vi "TalonFXSConfigurator.vi"(6 "timeoutSeconds":dbl=0.05, 8 "error in":errorcluster, 10 "DeviceConfiguration":T2={"Future Proof Configs"=FALSE, "MotorOutputInverted"=0, "MotorOutputNeutralMode"=0, "MotorOutputDutyCycleNeutralDeadband"=0.0, "MotorOutputPeakForwardDutyCycle"=1.0, "MotorOutputPeakReverseDutyCycle"=-1.0, "MotorOutputControlTimesyncFreqHz"=0.0, "CurrentLimitsStatorCurrentLimit"=120.0, "CurrentLimitsStatorCurrentLimitEnable"=TRUE, "CurrentLimitsSupplyCurrentLimit"=70.0, "CurrentLimitsSupplyCurrentLimitEnable"=TRUE, "CurrentLimitsSupplyCurrentLowerLimit"=40.0, "CurrentLimitsSupplyCurrentLowerTime"=1.0, "VoltageSupplyVoltageTimeConstant"=0.0, "VoltagePeakForwardVoltage"=16.0, "VoltagePeakReverseVoltage"=-16.0, "ExternalFeedbackSensorToMechanismRatio"=1.0, "ExternalFeedbackRotorToSensorRatio"=1.0, "ExternalFeedbackFeedbackRemoteSensorID"=0, "ExternalFeedbackVelocityFilterTimeConstant"=0.0, "ExternalFeedbackAbsoluteSensorOffset"=0.0, "ExternalFeedbackExternalFeedbackSensorSource"=0, "ExternalFeedbackSensorPhase"=0, "ExternalFeedbackQuadratureEdgesPerRotation"=4096, "ExternalFeedbackAbsoluteSensorDiscontinuityPoint"=0.5, "DifferentialSensorsDifferentialSensorSource"=0, "DifferentialSensorsDifferentialTalonFXSensorID"=0, "DifferentialSensorsDifferentialRemoteSensorID"=0, "DifferentialSensorsSensorToDifferentialRatio"=1.0, "DifferentialConstantsPeakDifferentialDutyCycle"=1.0, "DifferentialConstantsPeakDifferentialVoltage"=16.0, "DifferentialConstantsPeakDifferentialTorqueCurrent"=800.0, "OpenLoopRampsDutyCycleOpenLoopRampPeriod"=0.0, "OpenLoopRampsVoltageOpenLoopRampPeriod"=0.0, "OpenLoopRampsTorqueOpenLoopRampPeriod"=0.0, "ClosedLoopRampsDutyCycleClosedLoopRampPeriod"=0.0, "ClosedLoopRampsVoltageClosedLoopRampPeriod"=0.0, "ClosedLoopRampsTorqueClosedLoopRampPeriod"=0.0, "HardwareLimitSwitchForwardLimitType"=0, "HardwareLimitSwitchForwardLimitAutosetPositionEnable"=FALSE, "HardwareLimitSwitchForwardLimitAutosetPositionValue"=0.0, "HardwareLimitSwitchForwardLimitEnable"=TRUE, "HardwareLimitSwitchForwardLimitSource"=0, "HardwareLimitSwitchForwardLimitRemoteSensorID"=0, "HardwareLimitSwitchReverseLimitType"=0, "HardwareLimitSwitchReverseLimitAutosetPositionEnable"=FALSE, "HardwareLimitSwitchReverseLimitAutosetPositionValue"=0.0, "HardwareLimitSwitchReverseLimitEnable"=TRUE, "HardwareLimitSwitchReverseLimitSource"=0, "HardwareLimitSwitchReverseLimitRemoteSensorID"=0, "AudioBeepOnBoot"=TRUE, "AudioBeepOnConfig"=TRUE, "AudioAllowMusicDurDisable"=FALSE, "SoftwareLimitSwitchForwardSoftLimitEnable"=FALSE, "SoftwareLimitSwitchReverseSoftLimitEnable"=FALSE, "SoftwareLimitSwitchForwardSoftLimitThreshold"=0.0, "SoftwareLimitSwitchReverseSoftLimitThreshold"=0.0, "MotionMagicMotionMagicCruiseVelocity"=0.0, "MotionMagicMotionMagicAcceleration"=0.0, "MotionMagicMotionMagicJerk"=0.0, "MotionMagicMotionMagicExpo_kV"=0.12, "MotionMagicMotionMagicExpo_kA"=0.1, "CustomParamsCustomParam0"=0, "CustomParamsCustomParam1"=0, "ClosedLoopGeneralContinuousWrap"=FALSE, "ClosedLoopGeneralDifferentialContinuousWrap"=FALSE, "ClosedLoopGeneralGainSchedErrorThreshold"=0.0, "ClosedLoopGeneralGainSchedKpBehavior"=0, "CommutationAdvancedHallSupport"=0, "CommutationMotorArrangement"=0, "CommutationBrushedMotorWiring"=0, "CustomBrushlessMotorMotorKv"=500.0, "CustomBrushlessMotorPolePairCount"=1, "CustomBrushlessMotorHallDuringAB"=0, "CustomBrushlessMotorHallDuringAC"=0, "CustomBrushlessMotorHallCCWSelect"=FALSE, "CustomBrushlessMotorHallDirection"=FALSE, "ExternalTempThermistorMaxTemperature"=0.0, "ExternalTempThermistorBeta"=0.0, "ExternalTempThermistorR0"=0.0, "ExternalTempTempSensorRequired"=0, "Slot0kP"=0.0, "Slot0kI"=0.0, "Slot0kD"=0.0, "Slot0kS"=0.0, "Slot0kV"=0.0, "Slot0kA"=0.0, "Slot0kG"=0.0, "Slot0GravityType"=0, "Slot0StaticFeedforwardSign"=0, "Slot0GravityArmPositionOffset"=0.0, "Slot0GainSchedBehavior"=0, "Slot1kP"=0.0, "Slot1kI"=0.0, "Slot1kD"=0.0, "Slot1kS"=0.0, "Slot1kV"=0.0, "Slot1kA"=0.0, "Slot1kG"=0.0, "Slot1GravityType"=0, "Slot1StaticFeedforwardSign"=0, "Slot1GravityArmPositionOffset"=0.0, "Slot1GainSchedBehavior"=0, "Slot2kP"=0.0, "Slot2kI"=0.0, "Slot2kD"=0.0, "Slot2kS"=0.0, "Slot2kV"=0.0, "Slot2kA"=0.0, "Slot2kG"=0.0, "Slot2GravityType"=0, "Slot2StaticFeedforwardSign"=0, "Slot2GravityArmPositionOffset"=0.0, "Slot2GainSchedBehavior"=0} {"MotorOutputInverted" items=["CounterClockwise_Positive", "Clockwise_Positive"]; "MotorOutputNeutralMode" items=["Coast", "Brake"]; "ExternalFeedbackExternalFeedbackSensorSource" items=["Commutation", "RemoteCANcoder", "RemotePigeon2Yaw", "RemotePigeon2Pitch", "RemotePigeon2Roll", "FusedCANcoder", "SyncCANcoder", "Quadrature", "PulseWidth", "RemoteCANdiPWM1", "RemoteCANdiPWM2", "RemoteCANdiQuadrature", "FusedCANdiPWM1", "FusedCANdiPWM2", "FusedCANdiQuadrature", "SyncCANdiPWM1", "SyncCANdiPWM2"]; "ExternalFeedbackSensorPhase" items=["Aligned", "Opposed"]; "DifferentialSensorsDifferentialSensorSource" items=["Disabled", "RemoteTalonFX_HalfDiff", "RemotePigeon2Yaw", "RemotePigeon2Pitch", "RemotePigeon2Roll", "RemoteCANcoder", "RemoteCANdiPWM1", "RemoteCANdiPWM2", "RemoteCANdiQuadrature"]; "HardwareLimitSwitchForwardLimitType" items=["NormallyOpen", "NormallyClosed"]; "HardwareLimitSwitchForwardLimitSource" items=["LimitSwitchPin"=0, "RemoteTalonFX"=1, "RemoteCANifier"=2, "RemoteCANcoder"=4, "RemoteCANrange"=6, "RemoteCANdiS1"=7, "RemoteCANdiS2"=8, "Disabled"=3]; "HardwareLimitSwitchReverseLimitType" items=["NormallyOpen", "NormallyClosed"]; "HardwareLimitSwitchReverseLimitSource" items=["LimitSwitchPin"=0, "RemoteTalonFX"=1, "RemoteCANifier"=2, "RemoteCANcoder"=4, "RemoteCANrange"=6, "RemoteCANdiS1"=7, "RemoteCANdiS2"=8, "Disabled"=3]; "ClosedLoopGeneralGainSchedKpBehavior" items=["Continuous", "Discontinuous"]; "CommutationAdvancedHallSupport" items=["Disabled", "Enabled"]; "CommutationMotorArrangement" items=["Disabled"=0, "Minion_JST"=1, "Brushed_DC"=2, "NEO_JST"=5, "NEO550_JST"=6, "VORTEX_JST"=7, "Custom Brushless"=8]; "CommutationBrushedMotorWiring" items=["Leads_A_and_B", "Leads_A_and_C", "Leads_B_and_C"]; "ExternalTempTempSensorRequired" items=["Required", "Not_Required"]; "Slot0GravityType" items=["Elevator_Static", "Arm_Cosine"]; "Slot0StaticFeedforwardSign" items=["UseVelocitySign", "UseClosedLoopSign"]; "Slot0GainSchedBehavior" items=["Inactive", "ZeroOutput", "UseSlot0", "UseSlot1", "UseSlot2"]; "Slot1GravityType" items=["Elevator_Static", "Arm_Cosine"]; "Slot1StaticFeedforwardSign" items=["UseVelocitySign", "UseClosedLoopSign"]; "Slot1GainSchedBehavior" items=["Inactive", "ZeroOutput", "UseSlot0", "UseSlot1", "UseSlot2"]; "Slot2GravityType" items=["Elevator_Static", "Arm_Cosine"]; "Slot2StaticFeedforwardSign" items=["UseVelocitySign", "UseClosedLoopSign"]; "Slot2GainSchedBehavior" items=["Inactive", "ZeroOutput", "UseSlot0", "UseSlot1", "UseSlot2"]}, 11 "DeviceReference":T1) -> (0 "error out":errorcluster)   [LabVIEW 2025]
uses:
  <vilib>/Rock Robotics/WPI/ThirdParty/Phoenix6/DeviceReference.ctl
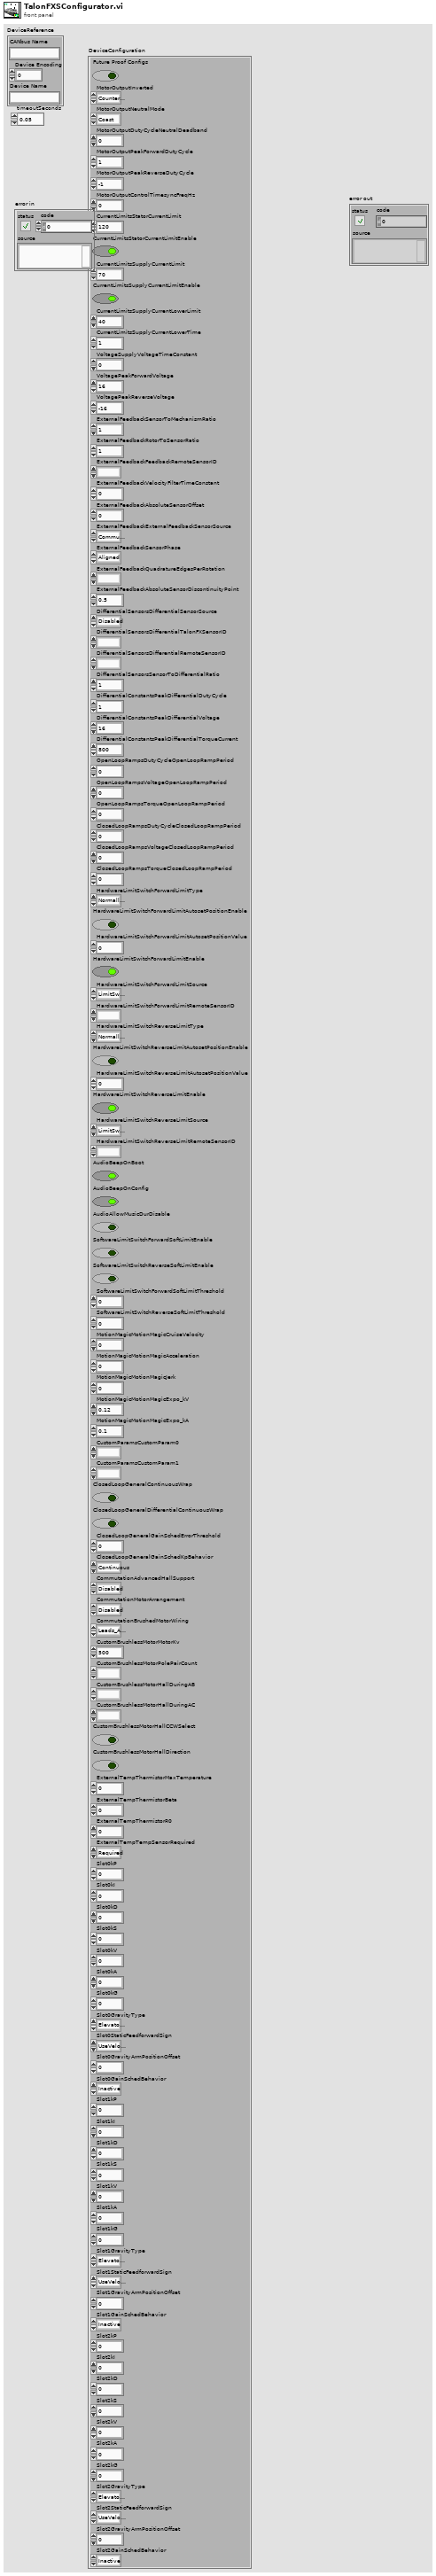
[diagram p1: front panel]
types:
  T1 = typedef "DeviceReference.ctl" = cluster{"CANbus Name":string, "Device Encoding":u32, "Device Name":string}
  T2 = cluster{"Future Proof Configs":bool, "MotorOutputInverted":u16, "MotorOutputNeutralMode":u16, "MotorOutputDutyCycleNeutralDeadband":dbl, "MotorOutputPeakForwardDutyCycle":dbl, "MotorOutputPeakReverseDutyCycle":dbl, "MotorOutputControlTimesyncFreqHz":dbl, "CurrentLimitsStatorCurrentLimit":dbl, "CurrentLimitsStatorCurrentLimitEnable":bool, "CurrentLimitsSupplyCurrentLimit":dbl, "CurrentLimitsSupplyCurrentLimitEnable":bool, "CurrentLimitsSupplyCurrentLowerLimit":dbl, "CurrentLimitsSupplyCurrentLowerTime":dbl, "VoltageSupplyVoltageTimeConstant":dbl, "VoltagePeakForwardVoltage":dbl, "VoltagePeakReverseVoltage":dbl, "ExternalFeedbackSensorToMechanismRatio":dbl, "ExternalFeedbackRotorToSensorRatio":dbl, "ExternalFeedbackFeedbackRemoteSensorID":u16, "ExternalFeedbackVelocityFilterTimeConstant":dbl, "ExternalFeedbackAbsoluteSensorOffset":dbl, "ExternalFeedbackExternalFeedbackSensorSource":u16, "ExternalFeedbackSensorPhase":u16, "ExternalFeedbackQuadratureEdgesPerRotation":u16, "ExternalFeedbackAbsoluteSensorDiscontinuityPoint":dbl, "DifferentialSensorsDifferentialSensorSource":u16, "DifferentialSensorsDifferentialTalonFXSensorID":u16, "DifferentialSensorsDifferentialRemoteSensorID":u16, "DifferentialSensorsSensorToDifferentialRatio":dbl, "DifferentialConstantsPeakDifferentialDutyCycle":dbl, "DifferentialConstantsPeakDifferentialVoltage":dbl, "DifferentialConstantsPeakDifferentialTorqueCurrent":dbl, "OpenLoopRampsDutyCycleOpenLoopRampPeriod":dbl, "OpenLoopRampsVoltageOpenLoopRampPeriod":dbl, "OpenLoopRampsTorqueOpenLoopRampPeriod":dbl, "ClosedLoopRampsDutyCycleClosedLoopRampPeriod":dbl, "ClosedLoopRampsVoltageClosedLoopRampPeriod":dbl, "ClosedLoopRampsTorqueClosedLoopRampPeriod":dbl, "HardwareLimitSwitchForwardLimitType":u16, "HardwareLimitSwitchForwardLimitAutosetPositionEnable":bool, "HardwareLimitSwitchForwardLimitAutosetPositionValue":dbl, "HardwareLimitSwitchForwardLimitEnable":bool, "HardwareLimitSwitchForwardLimitSource":u16, "HardwareLimitSwitchForwardLimitRemoteSensorID":u16, "HardwareLimitSwitchReverseLimitType":u16, "HardwareLimitSwitchReverseLimitAutosetPositionEnable":bool, "HardwareLimitSwitchReverseLimitAutosetPositionValue":dbl, "HardwareLimitSwitchReverseLimitEnable":bool, "HardwareLimitSwitchReverseLimitSource":u16, "HardwareLimitSwitchReverseLimitRemoteSensorID":u16, "AudioBeepOnBoot":bool, "AudioBeepOnConfig":bool, "AudioAllowMusicDurDisable":bool, "SoftwareLimitSwitchForwardSoftLimitEnable":bool, "SoftwareLimitSwitchReverseSoftLimitEnable":bool, "SoftwareLimitSwitchForwardSoftLimitThreshold":dbl, "SoftwareLimitSwitchReverseSoftLimitThreshold":dbl, "MotionMagicMotionMagicCruiseVelocity":dbl, "MotionMagicMotionMagicAcceleration":dbl, "MotionMagicMotionMagicJerk":dbl, "MotionMagicMotionMagicExpo_kV":dbl, "MotionMagicMotionMagicExpo_kA":dbl, "CustomParamsCustomParam0":u16, "CustomParamsCustomParam1":u16, "ClosedLoopGeneralContinuousWrap":bool, "ClosedLoopGeneralDifferentialContinuousWrap":bool, "ClosedLoopGeneralGainSchedErrorThreshold":dbl, "ClosedLoopGeneralGainSchedKpBehavior":u16, "CommutationAdvancedHallSupport":u16, "CommutationMotorArrangement":u16, "CommutationBrushedMotorWiring":u16, "CustomBrushlessMotorMotorKv":dbl, "CustomBrushlessMotorPolePairCount":u16, "CustomBrushlessMotorHallDuringAB":u16, "CustomBrushlessMotorHallDuringAC":u16, "CustomBrushlessMotorHallCCWSelect":bool, "CustomBrushlessMotorHallDirection":bool, "ExternalTempThermistorMaxTemperature":dbl, "ExternalTempThermistorBeta":dbl, "ExternalTempThermistorR0":dbl, "ExternalTempTempSensorRequired":u16, "Slot0kP":dbl, "Slot0kI":dbl, "Slot0kD":dbl, "Slot0kS":dbl, "Slot0kV":dbl, "Slot0kA":dbl, "Slot0kG":dbl, "Slot0GravityType":u16, "Slot0StaticFeedforwardSign":u16, "Slot0GravityArmPositionOffset":dbl, "Slot0GainSchedBehavior":u16, "Slot1kP":dbl, "Slot1kI":dbl, "Slot1kD":dbl, "Slot1kS":dbl, "Slot1kV":dbl, "Slot1kA":dbl, "Slot1kG":dbl, "Slot1GravityType":u16, "Slot1StaticFeedforwardSign":u16, "Slot1GravityArmPositionOffset":dbl, "Slot1GainSchedBehavior":u16, "Slot2kP":dbl, "Slot2kI":dbl, "Slot2kD":dbl, "Slot2kS":dbl, "Slot2kV":dbl, "Slot2kA":dbl, "Slot2kG":dbl, "Slot2GravityType":u16, "Slot2StaticFeedforwardSign":u16, "Slot2GravityArmPositionOffset":dbl, "Slot2GainSchedBehavior":u16}
  T3 = enum8{"<Null>", "I8", "I16", "I32", "I64", "U8", "U16", "U32", "U64", "SGL", "DBL", "EXT", "CSG", "CDB", "CXT", "0x0F", "0x10", "0x11", "0x12", "0x13", "0x14", "Enum U8", "Enum U16", "Enum U32", "Enum U64", "SGL PQ", "DBL PQ", "EXT PQ", "CSG PQ", "CDB PQ", "CXT PQ", "0x1F", "0x20", "Boolean", "0x22", "0x23", "0x24", "0x25", "0x26", "0x27", "0x28", "0x29", "0x2A", "0x2B", "0x2C", "0x2D", "0x2E", "0x2F", "String", "0x31", "Path", "Pict", "0x34", "0x35", "0x36", "DAQ", "0x38", "0x39", "0x3A", "0x3B", "0x3C", "0x3D", "0x3E", "0x3F", "Array", "0x41", "0x42", "0x43", "0x44", "0x45", "0x46", "0x47", "0x48", "0x49", "0x4A", "0x4B", "0x4C", "0x4D", "0x4E", "0x4F", "Cluster", "0x51", "0x52", "Variant", "Waveform", "0x55", "0x56", "0x57", "0x58", "0x59", "0x5A", "0x5B", "0x5C", "0x5D", "0x5E", "Fixed Point", "0x60", "0x61", "0x62", "0x63", "0x64", "0x65", "0x66", "0x67", "0x68", "0x69", "0x6A", "0x6B", "0x6C", "0x6D", "0x6E", "0x6F", "Refnum", "0x71", "0x72", "Set Collection", "Map Collection"}
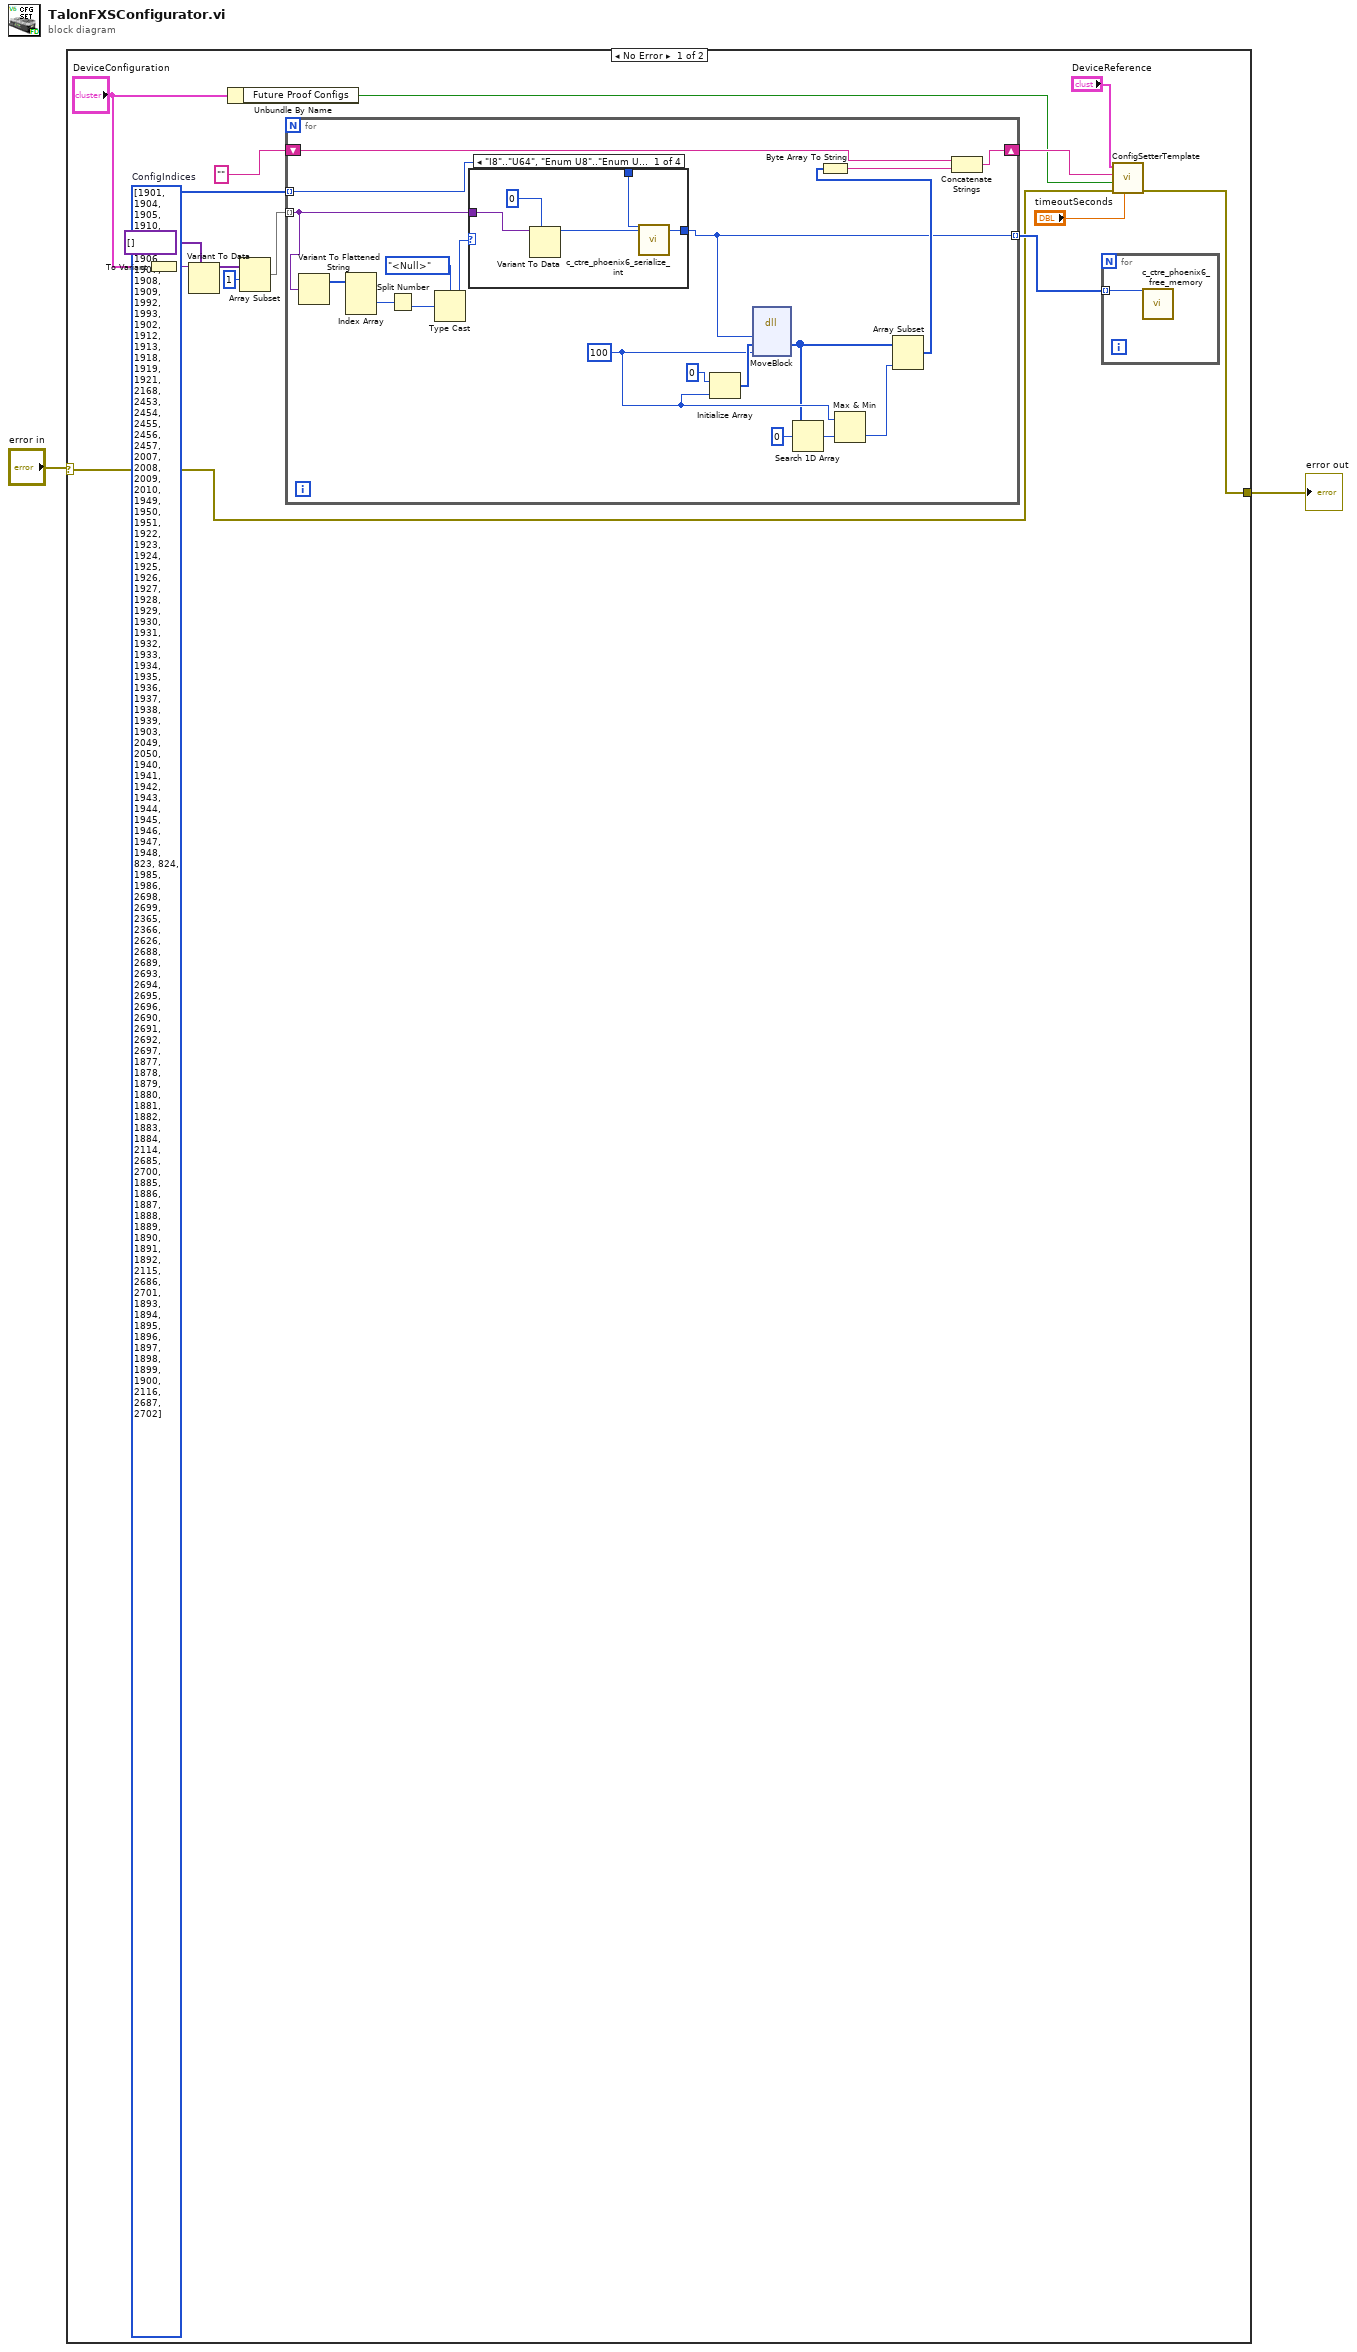
[diagram p0: block diagram]
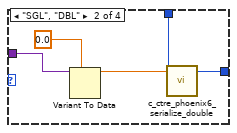
[diagram p2: hidden frame]
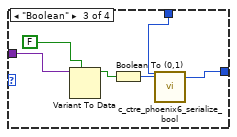
[diagram p3: hidden frame]
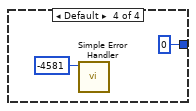
[diagram p4: hidden frame]
diagram:
  n1 = case shown="No Error" "error in" {
    selector: "error in" -> [w8 w56]
    tunnel: [w7 w56] -> w1
    frame No Error {
      w10 = i32[] [1901, 1904, 1905, 1910, 1911, 2167, 1906, 1907, 1908, 1909, 1992, 1993, 1902, 1912, 1913, 1918, 1919, 1921, 2168, 2453, 2454, 2455, 2456, 2457, 2007, 2008, 2009, 2010, 1949, 1950, 1951, 1922, 1923, 1924, 1925, 1926, 1927, 1928, 1929, 1930, 1931, 1932, 1933, 1934, 1935, 1936, 1937, 1938, 1939, 1903, 2049, 2050, 1940, 1941, 1942, 1943, 1944, 1945, 1946, 1947, 1948, 823, 824, 1985, 1986, 2698, 2699, 2365, 2366, 2626, 2688, 2689, 2693, 2694, 2695, 2696, 2690, 2691, 2692, 2697, 1877, 1878, 1879, 1880, 1881, 1882, 1883, 1884, 2114, 2685, 2700, 1885, 1886, 1887, 1888, 1889, 1890, 1891, 1892, 2115, 2686, 2701, 1893, 1894, 1895, 1896, 1897, 1898, 1899, 1900, 2116, 2687, 2702]  # ConfigIndices
      n2 = To Variant(anything="DeviceConfiguration") -> (Variant=w6:variant)
      n3 = Variant To Data(type=variant[] [], Variant=w6) -> (data=w3:variant[])  [unwired: 1 in, 1 out]
      n4 = Unbundle By Name("DeviceConfiguration") -> ("Future Proof Configs"=w9:bool)
      n5 = Array Subset(array=w3, index=1) -> (w12:variant[])  [unwired: 1 in]
      n6 = for {
        tunnel: w12 -> [w19] mode=indexing
        shift-right: [w35] -> w16
        shift-left: "" -> [w36]
        tunnel: [w24] -> w11 mode=indexing
        tunnel: w10 -> [w25] mode=indexing
        w28 = i64 100 ("size")
        n7 = Variant To Flattened String(Variant=w19) -> (1:w22:i16[])  [unwired: 1 out]
        n8 = Index Array(array=w22) -> (element #2=w23:i16)  [unwired: 3 in, 2 out]
        n9 = Split Number(x=w23) -> (lo(x)=w20:u8)  [unwired: 1 out]
        n10 = Type Cast(type=T3."<Null>", x=w20) -> (*(type *) &x=w18:T3)
        n11 = case shown="\"I8\"..\"U64\", \"Enum U8\"..\"Enum U64\"" w18 {
          tunnel: w19 -> [w41 w46 w52 _]
          tunnel: w25 -> [w39 w43 w48 _]
          tunnel: [w37 w42 w47 u32 0 ("Numeric 4")] -> w24
          frame "I8".."U64", "Enum U8".."Enum U64" {
            n12 = Variant To Data(type=0, Variant=w41) -> (data=w38:i32)  [unwired: 1 in, 1 out]
            n13 = call <vilib>:"c_ctre_phoenix6_serialize_int.vi"("Numeric 2"=w39, "Numeric 3"=w38) -> ("Numeric 4"=w37:u32)  [unwired: 24 in, 1 out]
          }
          frame "SGL", "DBL" {
            n14 = Variant To Data(type=0.0, Variant=w46) -> (data=w44:dbl)  [unwired: 1 in, 1 out]
            n15 = call <vilib>:"c_ctre_phoenix6_serialize_double.vi"("Numeric 2"=w43, "Numeric 3"=w44) -> ("Numeric 4"=w42:u32)  [unwired: 24 in, 1 out]
          }
          frame "Boolean" {
            n16 = Variant To Data(type=FALSE, Variant=w52) -> (data=w50:bool)  [unwired: 1 in, 1 out]
            n17 = Boolean To (0,1)(Boolean=w50) -> (0, 1=w49:i16)
            n18 = call <vilib>:"c_ctre_phoenix6_serialize_bool.vi"("Numeric 2"=w48, "Numeric 3"=w49) -> ("Numeric 4"=w47:u32)  [unwired: 24 in, 1 out]
          }
          frame Default {
            n19 = call <vilib>:"Simple Error Handler.vi"("error code (no error:0)"=-4581) -> ()  [unwired: 4 in, 5 out]
          }
        }
        n20 = Initialize Array(u8 0 ("element"), w28) -> (w33:u8[])
        n21 = dll-call lib="LabVIEW" fn="MoveBlock"("ps"=w24, "pd"=w33, "size"=w28) -> ("pd"=w27:u8[])  [unwired: 6 in, 2 out]
        n22 = Search 1D Array(1D array=w27, element=u8 0) -> (index of element=w29:i32)  [unwired: 1 in]
        n23 = Max & Min(x=w28, y=w29) -> (min(x,y)=w26:i64)  [unwired: 1 out]
        n24 = Array Subset(array=w27, length=w26) -> (w31:u8[])  [unwired: 1 in]
        n25 = Byte Array To String(unsigned byte array=w31) -> (string=w34:string)
        n26 = Concatenate Strings(w36, w34) -> (w35:string)
      }
      n27 = for {
        tunnel: w11 -> [w55] mode=indexing
        n28 = call <vilib>:"c_ctre_phoenix6_free_memory.vi"("Numeric 3"=w55) -> ()  [unwired: 25 in, 2 out]
      }
      n29 = call <vilib>:"ConfigSetterTemplate.vi"("timeoutSeconds"="timeoutSeconds", "error in"=w8, "FutureProofConfigs"=w9, "Configs"=w16, "DeviceReference"="DeviceReference") -> ("error out"=w7:errorcluster)  [unwired: 6 in]
    }
    frame Error {
    }
  }
  "error out" <- w1
